vi "sub_qam_symbol_map_gen.vi"(9 "Gray code?":bool, 11 "M-QAM":i32) -> (3 "symbol map":cdb[](array[numeric]))   [LabVIEW 2014]
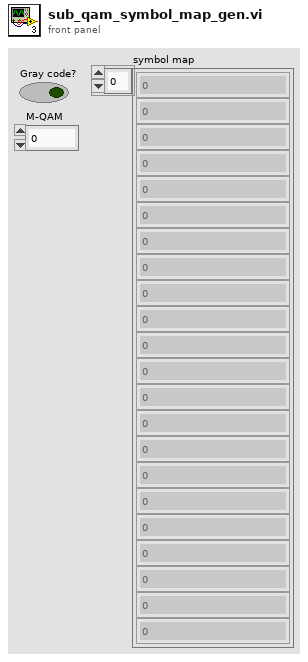
[diagram p1: front panel]
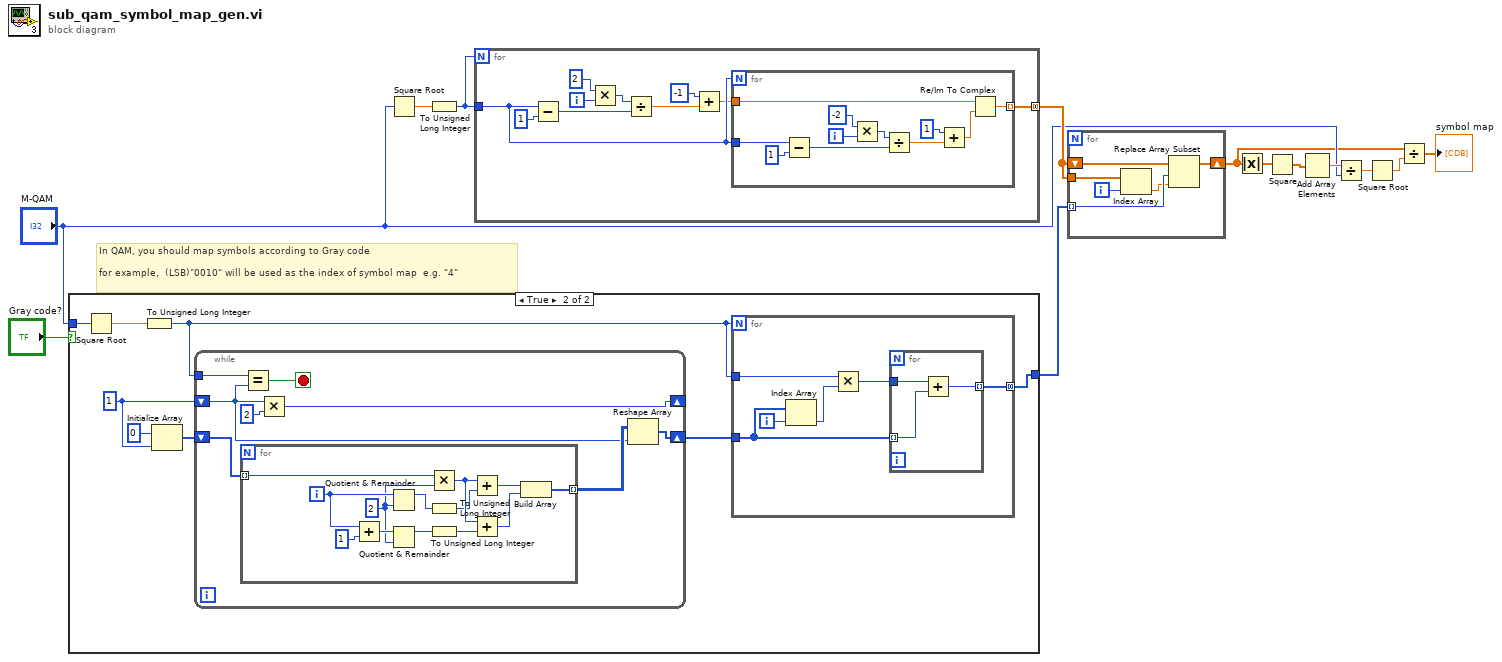
[diagram p0: block diagram]
diagram:
  # "In QAM, you should map symbols according to Gray code\n\nfor example,  (LSB)\"0010\" will be used as the index of symbol map  e.g. \"4\""
  n1 = case shown="True" "Gray code?" {
    tunnel: "M-QAM" -> [w15 w20]
    tunnel: [w14 w17] -> w10
    frame False {
      n2 = for {
        N: w15 -> [_]
        tunnel: [w16] -> w14 mode=indexing
        i -> [w16]
      }
    }
    frame True {
      w22 = u32 1
      n3 = Square Root(x=w20) -> (sqrt(x)=w21:dbl)
      n4 = To Unsigned Long Integer(number=w21) -> (unsigned 32bit integer=w18:u32)
      n5 = Initialize Array(u32 0, w22) -> (w23:u32[])
      n6 = while {
        tunnel: w18 -> [w39]
        shift-right: [w41] -> _
        shift-left: w22 -> [w35]
        shift-right: [w34] -> w19
        shift-left: w23 -> [w37]
        stop <- w38 stop-if-true
        n7 = for {
          tunnel: w37 -> [w54] mode=indexing
          tunnel: [w44] -> w36 mode=indexing
          i -> [w53]
          w50 = u32 2
          n8 = Add(x=w53, y=u32 1) -> (x+y=w51:u32)
          n9 = Quotient & Remainder(x=w53, y=w50) -> (x-y*floor(x/y)=w43:u32)  [unwired: 1 out]
          n10 = Quotient & Remainder(x=w51, y=w50) -> (x-y*floor(x/y)=w42:u32)  [unwired: 1 out]
          n11 = Multiply(x=w54, y=w50) -> (x*y=w47:u32)
          n12 = To Unsigned Long Integer(number=w43) -> (unsigned 32bit integer=w46:u32)
          n13 = To Unsigned Long Integer(number=w42) -> (unsigned 32bit integer=w45:u32)
          n14 = Add(x=w47, y=w46) -> (x+y=w49:u32)
          n15 = Add(x=w47, y=w45) -> (x+y=w48:u32)
          n16 = Build Array(w49, w48) -> (w44:u32[])
        }
        n17 = Equal?(x=w39, y=w35) -> (x = y?=w38:bool)
        n18 = Multiply(x=w35, y=u32 2) -> (x*y=w41:u32)
        n19 = Reshape Array(w36, w35) -> (w34:u32[])
      }
      n20 = for {
        N: w18 -> [_]
        tunnel: w19 -> [w27]
        tunnel: w18 -> [w28]
        tunnel: [w25] -> w17 mode=concatenating
        i -> [w30]
        n21 = Index Array(array=w27, index=w30) -> (element=w29:u32)
        n22 = Multiply(x=w28, y=w29) -> (x*y=w26:u32)
        n23 = for {
          tunnel: w27 -> [w32] mode=indexing
          tunnel: w26 -> [w33]
          tunnel: [w31] -> w25 mode=indexing
          n24 = Add(x=w33, y=w32) -> (x+y=w31:u32)
        }
      }
    }
  }
  n25 = Square Root(x="M-QAM") -> (sqrt(x)=w12:dbl)
  n26 = To Unsigned Long Integer(number=w12) -> (unsigned 32bit integer=w11:u32)
  n27 = for {
    N: w11 -> [_]
    tunnel: w11 -> [w57]
    tunnel: [w55] -> w9 mode=concatenating
    i -> [w62]
    n28 = Subtract(x=w57, y=u32 1) -> (x-y=w60:u32)
    n29 = Multiply(x=u32 2, y=w62) -> (x*y=w61:u32)
    n30 = Divide(x=w61, y=w60) -> (x/y=w59:dbl)
    n31 = Add(x=-1, y=w59) -> (x+y=w56:dbl)
    n32 = for {
      N: w57 -> [_]
      tunnel: w57 -> [w71]
      tunnel: w56 -> [w67]
      tunnel: [w65] -> w55 mode=indexing
      i -> [w69]
      n33 = Subtract(x=w71, y=u32 1) -> (x-y=w74:u32)
      n34 = Multiply(x=-2, y=w69) -> (x*y=w75:i32)
      n35 = Divide(x=w75, y=w74) -> (x/y=w73:dbl)
      n36 = Add(x=1, y=w73) -> (x+y=w66:dbl)
      n37 = Re/Im To Complex(1:w66, 2:w67) -> (0:w65:cdb)
    }
  }
  n38 = for {
    tunnel: w9 -> [w81]
    tunnel: w10 -> [w78] mode=indexing
    shift-right: [w79] -> w2
    shift-left: w9 -> [w80]
    i -> [w77]
    n39 = Index Array(array=w81, index=w77) -> (element=w76:cdb)
    n40 = Replace Array Subset(array=w80, new element=w76, index=w78) -> (w79:cdb[])
  }
  n41 = Absolute Value(x=w2) -> (abs(x)=w7:dbl[])
  n42 = Square(x=w7) -> (x^2=w6:dbl[])
  n43 = Add Array Elements(numeric array=w6) -> (sum=w8:dbl)
  n44 = Divide(x=w8, y="M-QAM") -> (x/y=w4:dbl)
  n45 = Square Root(x=w4) -> (sqrt(x)=w3:dbl)
  n46 = Divide(x=w2, y=w3) -> (x/y=→"symbol map":cdb[])
